vi "changeBit.vi"(9 "bit":bool, 10 "n":i32=-1, 11 "input":u8 format="%08b") -> (3 "output":u8 format="%08b")   [LabVIEW 2013, in "bitwiseOps.lvlib"]
uses:
  bitwiseOps.lvlib
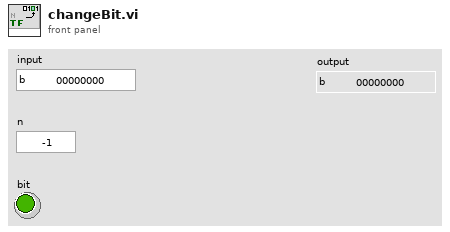
[diagram p1: front panel]
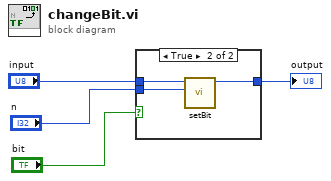
[diagram p0: block diagram]
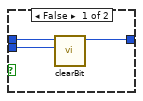
[diagram p2: hidden frame]
diagram:
  n1 = case shown="True" "bit" {
    tunnel: "input" -> [w7 w10]
    tunnel: "n" -> [w6 w9]
    tunnel: [w5 w8] -> w2
    frame False {
      n2 = call "clearBit.vi"("n"=w6, "input"=w7) -> ("output"=w5:u8)  [unwired: 9 in]
    }
    frame True {
      n3 = call "setBit.vi"("n"=w9, "input"=w10) -> ("output"=w8:u8)  [unwired: 9 in]
    }
  }
  "output" <- w2
